vi "PSTR-Fit Model.vi"(0 "PSTH":dbl[](array[numeric]), 7 "dt (ms)":dbl, 9 "delay (ms)":dbl, 11 "durat (ms)":dbl) -> (4 "Fit":T1)   [LabVIEW 2020]
uses:
  Typedefs/PSTR-Model Fit.ctl
  Typedefs/PSTR-Fit Parameters.ctl
  epl-vi-lib/Utility VIs/Math VIs/LinSpace (x0-dx-npts).vi
  <vilib>/Analysis/baseanly.llb/Mean (DBL).vi
  <vilib>/gmath/NumericalOptimization/Nonlinear Curve Fit LM bound.vi
  <vilib>/gmath/NI_Gmath.lvlib
  <vilib>/Analysis/NI_AALBase.lvlib
panel:
  out "latency":dbl
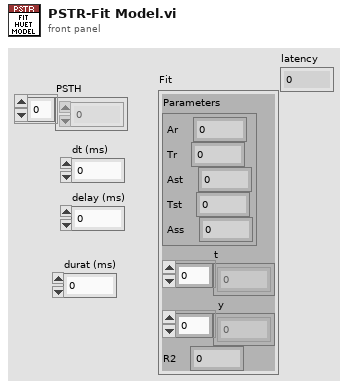
[diagram p1: front panel]
types:
  T1 = typedef "PSTR-Model Fit.ctl" = cluster{"Parameters":T2, "t":dbl[], "y":dbl[], "R2":dbl}
  T2 = typedef "PSTR-Fit Parameters.ctl" = cluster{"Ar":dbl, "Tr":dbl, "Ast":dbl, "Tst":dbl, "Ass":dbl}
  T3 = cluster{"best fit parameters[0]":dbl, "best fit parameters[1]":dbl, "best fit parameters[2]":dbl, "best fit parameters[3]":dbl, "best fit parameters[4]":dbl}
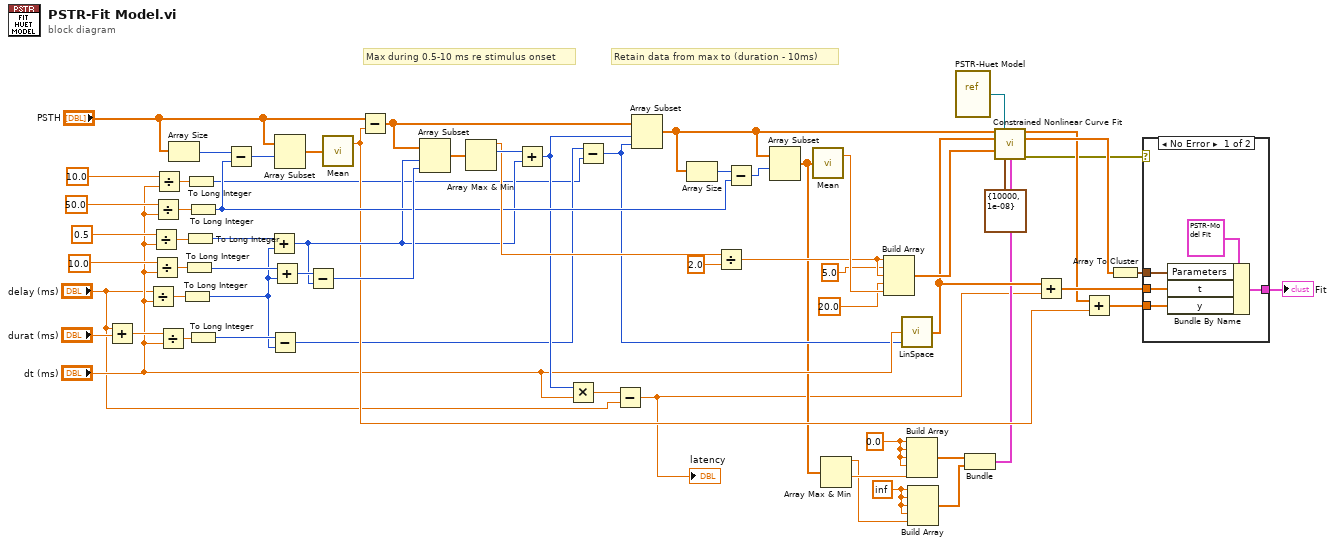
[diagram p0: block diagram]
diagram:
  w8 = inf ("Numeric")
  w11 = 0.0 ("Numeric")
  # "Retain data from max to (duration - 10ms)"
  # "Max during 0.5-10 ms re stimulus onset"
  n1 = Add(x="delay (ms)", y="durat (ms)") -> (x+y=w61:dbl)
  n2 = Divide(x="delay (ms)", y="dt (ms)") -> (x/y=w63:dbl)
  n3 = Divide(x=0.5, y="dt (ms)") -> (x/y=w57:dbl)
  n4 = Divide(x=10.0, y="dt (ms)") -> (x/y=w56:dbl)
  n5 = Divide(x=50.0, y="dt (ms)") -> (x/y=w47:dbl)
  n6 = Divide(x=10.0, y="dt (ms)") -> (x/y=w14:dbl)
  n7 = Divide(x=w61, y="dt (ms)") -> (x/y=w60:dbl)
  n8 = Array Size(array="PSTH") -> (size(s)=w45:i32)
  n9 = To Long Integer(number=w63) -> (32bit integer=w49:i32)
  n10 = To Long Integer(number=w56) -> (32bit integer=w55:i32)
  n11 = To Long Integer(number=w57) -> (32bit integer=w17:i32)
  n12 = To Long Integer(number=w14) -> (32bit integer=w13:i32)
  n13 = To Long Integer(number=w47) -> (32bit integer=w31:i32)
  n14 = To Long Integer(number=w60) -> (32bit integer=w50:i32)
  n15 = Subtract(x=w45, y=w31) -> (x-y=w41:i32)
  n16 = Add(x=w17, y=w49) -> (x+y=w29:i32)
  n17 = Subtract(x=w50, y=w49) -> (x-y=w18:i32)
  n18 = Add(x=w55, y=w49) -> (x+y=w51:i32)
  n19 = Array Subset(array="PSTH", index=w41) -> (w44:dbl[])  [unwired: 1 in]
  n20 = Subtract(x=w51, y=w29) -> (x-y=w54:i32)
  n21 = call-poly <vilib>:"Mean.vi"("X"=w44) -> ("mean"=w22:dbl)  [unwired: 1 out]
  n22 = Subtract(x="PSTH", y=w22) -> (x-y=w43:dbl[])
  n23 = Array Subset(array=w43, index=w29, length=w54) -> (w53:dbl[])
  n24 = Array Max & Min(array=w53) -> (max value=w38:dbl, max index (indices)=w52:i32)  [unwired: 2 out]
  n25 = Add(x=w52, y=w29) -> (x+y=w24:i32)
  n26 = Multiply(x=w24, y="dt (ms)") -> (x*y=w3:dbl)
  n27 = Subtract(x=w18, y=w13) -> (x-y=w12:i32)
  n28 = Subtract(x=w3, y="delay (ms)") -> (x-y=w2:dbl)
  "latency" <- w2
  n29 = Array Subset(array=w43, index=w24, length=w12) -> (w30:dbl[])
  n30 = Array Size(array=w30) -> (size(s)=w33:i32)
  n31 = Divide(x=w38, y=2.0) -> (x/y=w36:dbl)
  n32 = Subtract(x=w33, y=w31) -> (x-y=w32:i32)
  n33 = Array Subset(array=w30, index=w32) -> (w6:dbl[])  [unwired: 1 in]
  n34 = call-poly <vilib>:"Mean.vi"("X"=w6) -> ("mean"=w40:dbl)  [unwired: 1 out]
  n35 = Array Max & Min(array=w6) -> (max value=w4:dbl, min value=w5:dbl)  [unwired: 2 out]
  n36 = Build Array(w36, 5.0, w36, 20.0 ("x/y"), w40) -> (w39:dbl[])
  n37 = call-poly "LinSpace.vi"("npts"=w12, "dx"="dt (ms)") -> ("Array"=w26:dbl[])  [unwired: 2 in, 1 out]
  n38 = Build Array(w11, w11, w11, w11, w5) -> (w10:dbl[])
  n39 = Build Array(w8, w8, w8, w8, w4) -> (w7:dbl[])
  n40 = vi-ref "PSTR-Huet Model.vi"() -> (w42:refnum<vi>)
  n41 = Bundle(w10, w7) -> (w9:cluster{dbl[], dbl[]})  [unwired: 1 in]
  n42 = call-poly <vilib>:"Constrained Nonlinear Curve Fit.vi"("Y"=w30, "f(x,a)"=w42, "X"=w26, "initial parameters"=w39, "termination"=cluster{"max iteration":i32, "tolerance":dbl} {"max iteration"=10000, "tolerance"=1e-08}, "parameter bounds"=w9) -> ("best nonlinear fit"=w23:dbl[], "best fit parameters"=w28:dbl[], "error out"=w19:errorcluster)  [unwired: 4 in, 3 out]
  n43 = Add(x=w26, y=w2) -> (x+y=w25:dbl[])
  n44 = Add(x=w23, y=w22) -> (x+y=w21:dbl[])
  n45 = Array To Cluster(array=w28) -> (cluster=w27:T3)
  n46 = case shown="No Error" w19 {
    tunnel: w27 -> [w68 _]
    tunnel: w25 -> [w67 _]
    tunnel: w21 -> [w66 _]
    tunnel: [w65 _] -> w20
    frame No Error {
      n47 = Bundle By Name(cluster=T1 {"Parameters"={"Ar"=0.0, "Tr"=0.0, "Ast"=0.0, "Tst"=0.0, "Ass"=0.0}, "t"=[], "y"=[], "R2"=0.0} ("Fit"), "Parameters"=w68, "t"=w67, "y"=w66) -> (w65:T1)
    }
    frame Error {
    }
  }
  "Fit" <- w20
